vi "File updated.vi"(8 "error in (no error)":errorcluster, 10 "File Path Control":path, 11 "MagLabGraph in":refnum<class "MagLabGraph.lvclass">) -> (0 "error out":errorcluster, 3 "MagLabGraph out":refnum<class "MagLabGraph.lvclass">)   [LabVIEW 2015, in "MagLabGraph.lvclass"]
uses:
  MagLabGraph.lvclass
  <vilib>/ActorFramework/Actor/Actor.lvclass/Actor.ctl
  <vilib>/ActorFramework/Message Enqueuer/Message Enqueuer.lvclass/Message Enqueuer.ctl
  MagLabGraph.lvclass/MagLabGraph.ctl
  <vilib>/ActorFramework/Message Enqueuer/Init from Existing Queue.vi
  <vilib>/ActorFramework/Message Enqueuer/Enqueue.vi
  <vilib>/ActorFramework/Message Priority Queue/Priority Enqueue.vi
  <vilib>/ActorFramework/Message Enqueuer/Message Enqueuer.lvclass
  MagLabGraph Messages/Replot Msg/Replot Msg.lvclass
  <vilib>/ActorFramework/Actor/Actor.lvclass
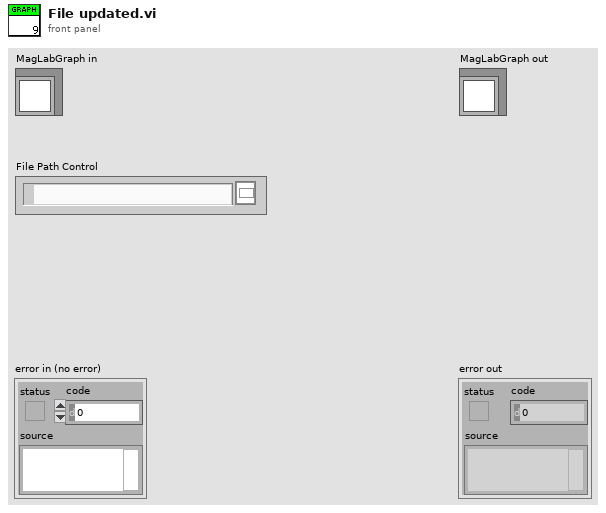
[diagram p1: front panel]
types:
  T1 = cluster{"File Path Control":path, "Group":string, "Channel":string, "Abbreviated":string}[]
  T2 = cluster{"File Path Control":path, "Group":string, "Channel":string, "Abbreviated":string}
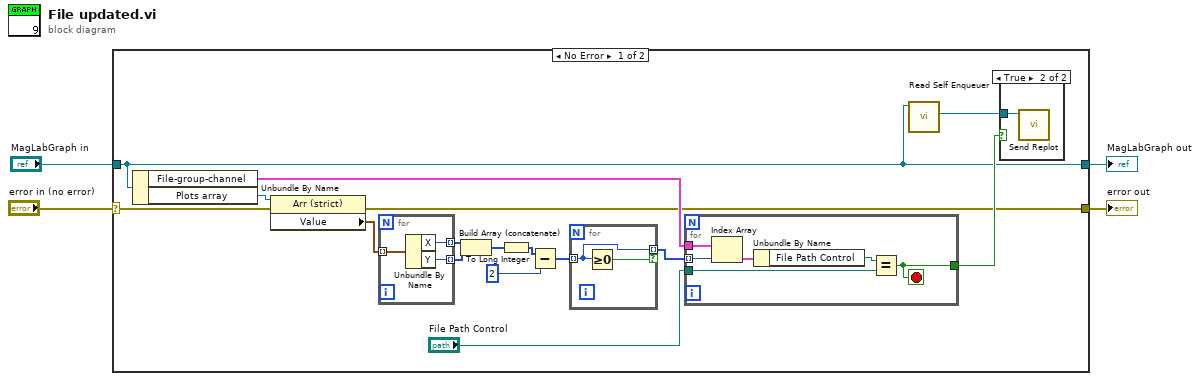
[diagram p0: block diagram]
diagram:
  n1 = case shown="No Error" "error in (no error)" {
    selector: "error in (no error)" -> [w11 w34]
    tunnel: [w10 w34] -> w3
    tunnel: [w13 w33] -> w1
    tunnel: "MagLabGraph in" -> [w13 w33]
    frame No Error {
      n2 = Unbundle By Name(w13) -> ("File-group-channel"=w16:T1, "Plots array"=w20:refnum<vi>)
      n3 = property class="Arr (strict)"(reference=w20, error in=w11) -> (error out=w10:errorcluster, "Value"=w19:cluster{"X":u16, "Y":u16}[])  [unwired: 1 out]
      n4 = for {
        tunnel: w19 -> [w32] mode=indexing
        tunnel: [w31] -> w18 mode=indexing
        tunnel: [w30] -> w17 mode=indexing
        n5 = Unbundle By Name(w32) -> ("X"=w31:u16, "Y"=w30:u16)
      }
      n6 = Build Array (concatenate)(w18, w17) -> (w9:u16[])
      n7 = To Long Integer(number=w9) -> (32bit integer=w7:i32[])
      n8 = Subtract(x=w7, y=2) -> (x-y=w6:i32[])
      n9 = for {
        tunnel: w6 -> [w22] mode=indexing
        tunnel: [w22] -> w5 mode=indexing if=w21
        n10 = Greater Or Equal To 0?(x=w22) -> (x >= 0?=w21:bool)
      }
      n11 = for {
        tunnel: w5 -> [w28] mode=indexing
        tunnel: w16 -> [w29]
        tunnel: "File Path Control" -> [w25]
        tunnel: [w24] -> w14
        stop <- w24 stop-if-true
        n12 = Index Array(array=w29, index=w28) -> (element=w27:T2)
        n13 = Unbundle By Name(w27) -> ("File Path Control"=w26:path)
        n14 = Equal?(x=w26, y=w25) -> (x = y?=w24:bool)
      }
      n15 = call <vilib>:"Read Self Enqueuer.vi"("Actor"=w13) -> ("Self Enqueuer"=w12:refnum<class "Message Enqueuer.lvclass">)  [unwired: 10 in]
      n16 = case shown="True" w14 {
        tunnel: w12 -> [_ w23]
        frame False {
        }
        frame True {
          n17 = call "Send Replot.vi"("Message Enqueuer"=w23) -> ()  [unwired: 9 in, 2 out]
        }
      }
    }
    frame Error {
    }
  }
  "error out" <- w3
  "MagLabGraph out" <- w1
